vi "GetImageIndex.vi"(9 "Supported Devices":u32[](array[numeric]), 10 "TargetInfoHistory":T1={"USBTargetList"={"TargetList"=[], "Value"=-1, "Target RT Info List"=[]}, "WiFiTargetList"={"TargetList"=[], "Value"=-1, "Target RT Info List"=[]}, "GenericTargetList"={"TargetList"=[], "Value"=-1, "Target RT Info List"=[]}, "IPTargetList"={"IP Error Out"={"status"=FALSE, "code"=0, "source"=""}, "Target RT Info List"=[]}} {"IPTargetList"."Target RT Info List"."ProdID" format="%.0x"; "USBTargetList"."Target RT Info List"."ProdID" format="%.0x"; "WiFiTargetList"."Target RT Info List"."ProdID" format="%.0x"; "GenericTargetList"."Target RT Info List"."ProdID" format="%.0x"}, 11 "AvailableTarget":T4) -> (3 "ProdID":u32)   [LabVIEW 2021, in "myRIOMetaDataObj.lvclass"]
uses:
  myRIOMetaDataObj.lvclass
  AvailableTargets.ctl
  TargetInfoHistory.ctl
  TargetListInfo.ctl
  <resource>/myRIO/Target Info.ctl
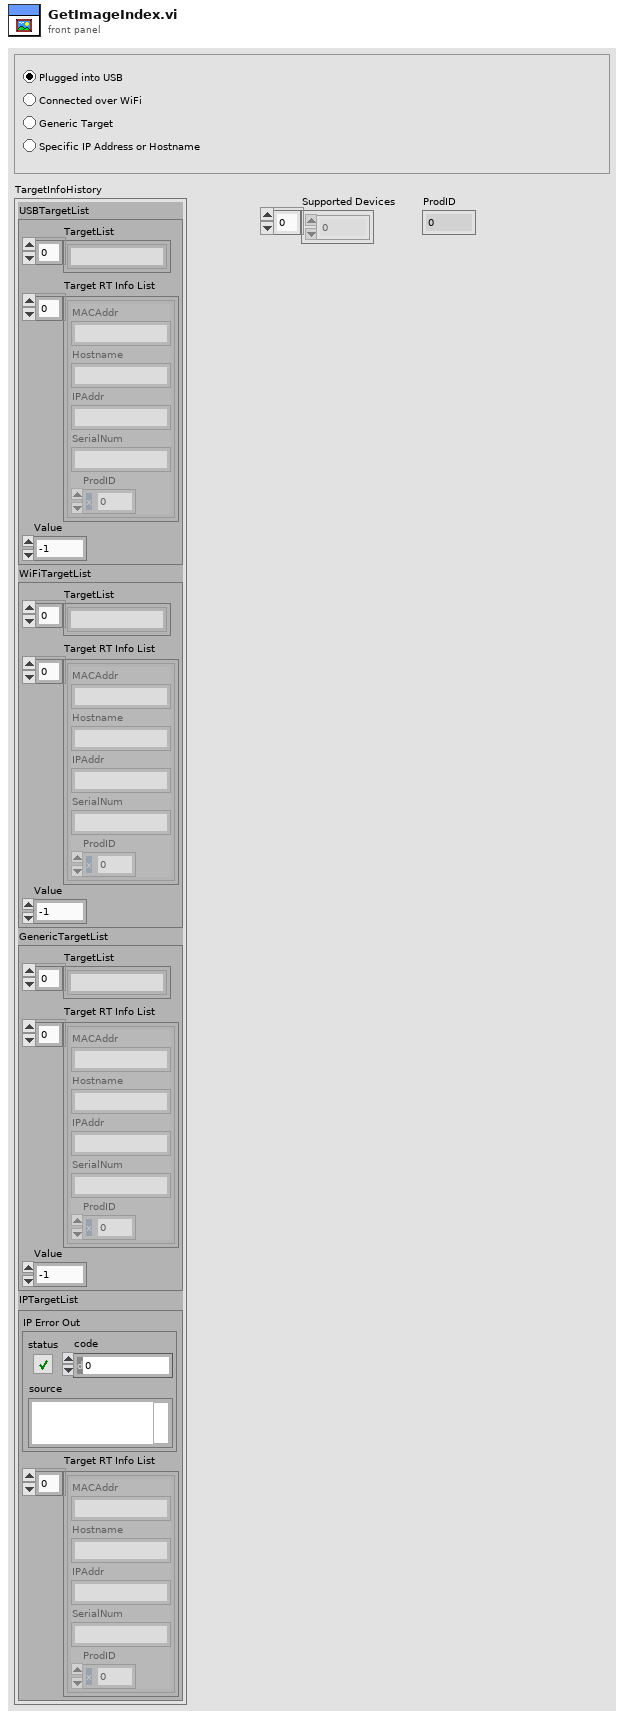
[diagram p1: front panel]
types:
  T1 = typedef "myRIOMetaDataObj.lvclass/TargetInfoHistory.ctl" = cluster{"USBTargetList":T2, "WiFiTargetList":T2, "GenericTargetList":T2, "IPTargetList":cluster{"IP Error Out":errorcluster, "Target RT Info List":T3[]}}
  T2 = typedef "myRIOMetaDataObj.lvclass/TargetListInfo.ctl" = cluster{"TargetList":string[], "Value":i32, "Target RT Info List":T3[]}
  T3 = typedef "Target Info.ctl" = cluster{"MACAddr":string, "Hostname":string, "IPAddr":string, "SerialNum":string, "ProdID":u32}
  T4 = typedef "myRIOMetaDataObj.lvclass/AvailableTargets.ctl" = enum32{"USBTarget", "WifiTarget", "NoSpecificTarget", "TargetIP"}
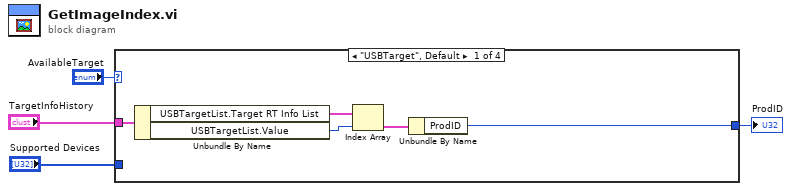
[diagram p0: block diagram]
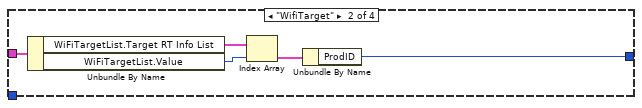
[diagram p2: hidden frame]
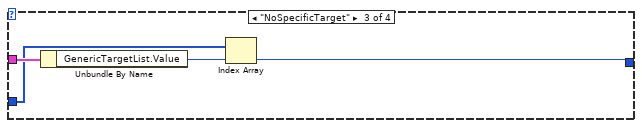
[diagram p3: hidden frame]
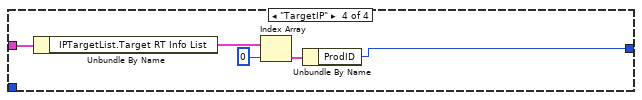
[diagram p4: hidden frame]
diagram:
  n1 = case shown="\"USBTarget\", Default" "AvailableTarget" {
    tunnel: "TargetInfoHistory" -> [w9 w11 w18 w23]
    tunnel: [w5 w10 w15 w19] -> w1
    tunnel: "Supported Devices" -> [_ _ w16 _]
    frame "USBTarget", Default {
      n2 = Unbundle By Name(w9) -> ("USBTargetList.Target RT Info List"=w8:T3[], "USBTargetList.Value"=w7:i32)
      n3 = Index Array(array=w8, index=w7) -> (element=w6:T3)
      n4 = Unbundle By Name(w6) -> ("ProdID"=w5:u32)
    }
    frame "WifiTarget" {
      n5 = Unbundle By Name(w11) -> ("WiFiTargetList.Target RT Info List"=w14:T3[], "WiFiTargetList.Value"=w13:i32)
      n6 = Index Array(array=w14, index=w13) -> (element=w12:T3)
      n7 = Unbundle By Name(w12) -> ("ProdID"=w10:u32)
    }
    frame "NoSpecificTarget" {
      n8 = Unbundle By Name(w18) -> ("GenericTargetList.Value"=w17:i32)
      n9 = Index Array(array=w16, index=w17) -> (element=w15:u32)
    }
    frame "TargetIP" {
      n10 = Unbundle By Name(w23) -> ("IPTargetList.Target RT Info List"=w21:T3[])
      n11 = Index Array(array=w21, index=0) -> (element=w22:T3)
      n12 = Unbundle By Name(w22) -> ("ProdID"=w19:u32)
    }
  }
  "ProdID" <- w1
